vi "Is Error.vi"(8 "Error In":errorcluster) -> (0 "Error Out":errorcluster)   [LabVIEW 2017, in "Tests.lvlib" / "Writer.lvlib"]
uses:
  Writer.lvlib
  src/LabPack/Public/Writer/Writer.lvclass/Writer.ctl
  src/LabPack/Public/Writer/Writer.lvclass
  <vilib>/addons/_JKI Toolkits/Caraya/classes/Test/Test.lvclass
  <vilib>/addons/_JKI Toolkits/Caraya/classes/Assert/Assert.lvclass
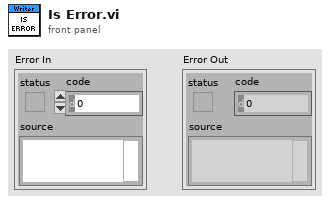
[diagram p1: front panel]
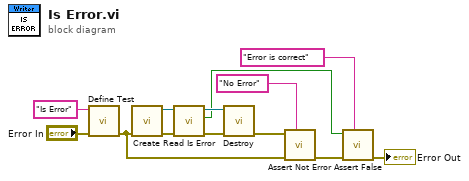
[diagram p0: block diagram]
diagram:
  n1 = call <vilib>:"Define Test.vi"("error in (no error)"="Error In", "Label (VI Title)"="Is Error") -> ("error out"=w9:errorcluster)  [unwired: 9 in]
  n2 = call "Create.vi"("Error In"=w9) -> ("Error Out"=w4:errorcluster, "Writer"=w7:refnum<class "Writer.lvclass">)  [unwired: 9 in]
  n3 = call "Read Is Error.vi"("Error In"=w4, "Writer In"=w7) -> ("Error Out"=w5:errorcluster, "Error"=w1:bool, "Writer Out"=w6:refnum<class "Writer.lvclass">)  [unwired: 7 in]
  n4 = call "Destroy.vi"("Error In"=w5, "Writer"=w6) -> ("Error Out"=w8:errorcluster)  [unwired: 9 in]
  n5 = call <vilib>:"Assert Not Error.vi"("Label"="No Error", "error in (no error)"=w9, "Not Error?"=w8) -> ("error out"=w11:errorcluster)  [unwired: 8 in]
  n6 = call <vilib>:"Assert False.vi"("Label"="Error is correct", "error in (no error)"=w11, "False?"=w1) -> ("error out"=→"Error Out":errorcluster)  [unwired: 8 in]
